vi "ArmPathPlanPreview.vi"(0 "RobotDimensions":T2, 2 "AvoidancePolygon":T6, 3 "Arm Pass Through Params":T1) -> (5 "Shoulder Path":T4[](array[typedef]) {"Time (ms)" items=["TrajectoryDuration_0ms"=0, "TrajectoryDuration_5ms"=5, "TrajectoryDuration_10ms"=10, "TrajectoryDuration_20ms"=20, "TrajectoryDuration_30ms"=30, "TrajectoryDuration_40ms"=40, "TrajectoryDuration_50ms"=50, "TrajectoryDuration_100ms"=100]}, 6 "Extension Path":T4[](array[typedef]) {"Time (ms)" items=["TrajectoryDuration_0ms"=0, "TrajectoryDuration_5ms"=5, "TrajectoryDuration_10ms"=10, "TrajectoryDuration_20ms"=20, "TrajectoryDuration_30ms"=30, "TrajectoryDuration_40ms"=40, "TrajectoryDuration_50ms"=50, "TrajectoryDuration_100ms"=100]}, 7 "Wrist Path":T4[](array[typedef]) {"Time (ms)" items=["TrajectoryDuration_0ms"=0, "TrajectoryDuration_5ms"=5, "TrajectoryDuration_10ms"=10, "TrajectoryDuration_20ms"=20, "TrajectoryDuration_30ms"=30, "TrajectoryDuration_40ms"=40, "TrajectoryDuration_50ms"=50, "TrajectoryDuration_100ms"=100]}, 8 "Go":bool)   [LabVIEW 2018]
uses:
  TypeDefs/ArmAbsolutePosition.ctl
  General/MotionProfiling/TypeDefs/MotionProfileGeneratorParams.ctl
  <vilib>/Rock Robotics/WPI/ThirdParty/Phoenix-LabVIEW/Motor Controller/Controls/CTRE_Phoenix_MotorControl_TrajectoryPointTimeDur.ctl
  General/MotionProfiling/TypeDefs/TrajectoryPoint.ctl
  ArgosLib/Path Planning/TypeDefs/Polygon2D.ctl
  ArgosLib/Path Planning/TypeDefs/Point2D.ctl
  TypeDefs/ConfigComponents/Config_Dimensions.ctl
  TypeDefs/ArmPassThroughParams.ctl
  ArgosLib/Signal Processing/TypeDefs/EdgeDetector_Type.ctl
  ArgosLib/ArgosLib.lvlib
panel:
  out "Wrist Path Graph":T3(graph)
  out "Shoulder Path Graph":T3(graph)
  in  "Preview?":bool
  in  "Send Path Plan":bool
  out "Extension Path Graph":T3(graph)
  in  "Reverse Direction":bool
  in  "MotionProfileGeneratorParameters":T8={"Trajectory Point Interval (ms)"=40, "Maximum Travel Speed (units/s)"=20.0, "Velocity Ramp Time (ms)"=400.0, "Acceleration Ramp Time (ms)"=200.0} {"Acceleration Ramp Time (ms)" min=1.0; "Velocity Ramp Time (ms)" min=1.0; "Maximum Travel Speed (units/s)" min=0.0; "Trajectory Point Interval (ms)" items=["TrajectoryDuration_0ms"=0, "TrajectoryDuration_5ms"=5, "TrajectoryDuration_10ms"=10, "TrajectoryDuration_20ms"=20, "TrajectoryDuration_30ms"=30, "TrajectoryDuration_40ms"=40, "TrajectoryDuration_50ms"=50, "TrajectoryDuration_100ms"=100]}
  in  "EndPoint":T9={"X (in)"=-21.5, "Y (in)"=0.0, "Wrist (rad)"=-1.57}
  in  "StartPoint":T9={"X (in)"=21.5, "Y (in)"=0.0, "Wrist (rad)"=1.57}
  in  "PathPointSpacing (in)":dbl=0.25
  in  "MaxArmLength":dbl=35.0
  in  "MinArmLength":dbl=17.0
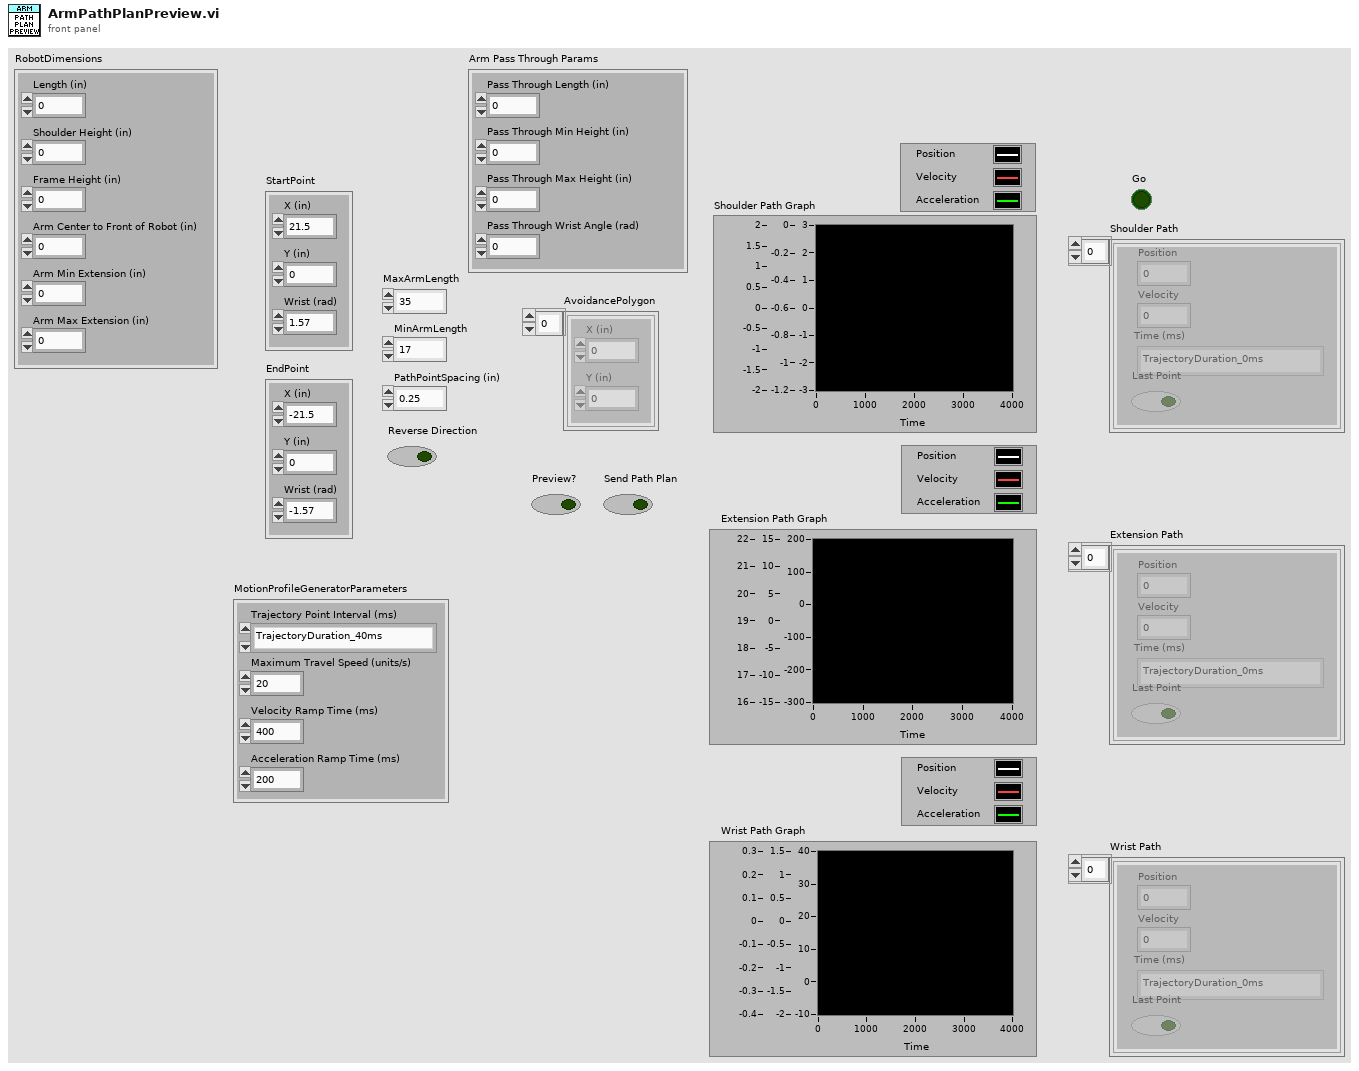
[diagram p1: front panel]
types:
  T1 = typedef "ArmPassThroughParams.ctl" = cluster{"Pass Through Length (in)":dbl, "Pass Through Min Height (in)":dbl, "Pass Through Max Height (in)":dbl, "Pass Through Wrist Angle (rad)":dbl}
  T2 = typedef "Config_Dimensions.ctl" = cluster{"Length (in)":dbl, "Shoulder Height (in)":dbl, "Frame Height (in)":dbl, "Arm Center to Front of Robot (in)":dbl, "Arm Min Extension (in)":dbl, "Arm Max Extension (in)":dbl}
  T3 = cluster{dbl, "Trajectory Point Interval (ms)":i32, dbl[][]}
  T4 = typedef "TrajectoryPoint.ctl" = cluster{"Position ":dbl, "Velocity ":dbl, "Time (ms)":T5, "Last Point":bool}
  T5 = typedef "CTRE_Phoenix_MotorControl_TrajectoryPointTimeDur.ctl" = i32
  T6 = typedef "ArgosLib.lvlib/Polygon2D.ctl" = T7[]
  T7 = typedef "ArgosLib.lvlib/Point2D.ctl" = cluster{"X (in)":dbl, "Y (in)":dbl}
  T8 = typedef "MotionProfileGeneratorParams.ctl" = cluster{"Trajectory Point Interval (ms)":T5, "Maximum Travel Speed (units/s)":dbl, "Velocity Ramp Time (ms)":dbl, "Acceleration Ramp Time (ms)":dbl}
  T9 = typedef "ArmAbsolutePosition.ctl" = cluster{"X (in)":dbl, "Y (in)":dbl, "Wrist (rad)":dbl}
  T10 = typedef "ArgosLib.lvlib/EdgeDetector_Type.ctl" = enum16{"RisingEdge", "FallingEdge", "Both"}
  T11 = cluster{dbl, "Trajectory Point Interval (ms)":T5, dbl[][]}
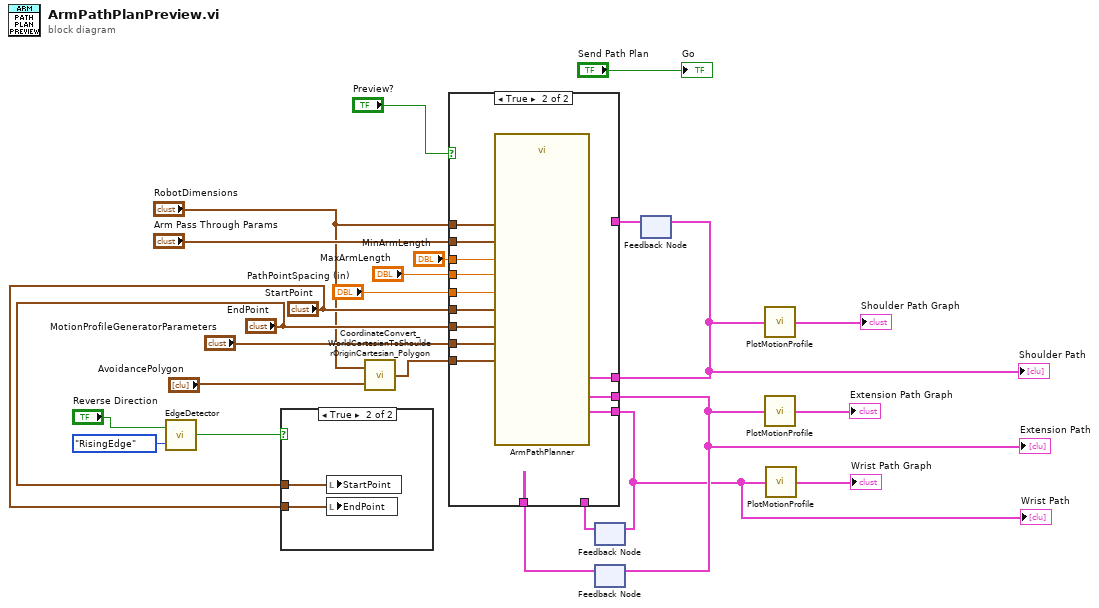
[diagram p0: block diagram]
diagram:
  n1 = call "EdgeDetector.vi"("DetectorType"=EdgeDetector_Type."RisingEdge", "Input"="Reverse Direction") -> ("Edge"=w20:bool)
  n2 = case shown="True" w20 {
    tunnel: "StartPoint" -> [_ w26]
    tunnel: "EndPoint" -> [_ w25]
    frame False {
    }
    frame True {
      n3 = local write "StartPoint"(w25) -> ()
      n4 = local write "EndPoint"(w26) -> ()
    }
  }
  n5 = call "CoordinateConvert_WorldCartesianToShoulderOriginCartesian_Polygon.vi"("ArmPositionIn"="AvoidancePolygon", "RobotDimensions"="RobotDimensions") -> ("ArmPositionRelativeToShoulder"=w2:T6)
  n6 = feedback #1() -> (w4:T4[])  [unwired: 1 in]
  n7 = feedback #2() -> (w11:T4[])  [unwired: 1 in]
  n8 = feedback #3() -> (w9:T4[])  [unwired: 1 in]
  n9 = case shown="True" "Preview?" {
    tunnel: "MinArmLength" -> [_ w41]
    tunnel: "MaxArmLength" -> [_ w40]
    tunnel: "PathPointSpacing (in)" -> [_ w39]
    tunnel: "MotionProfileGeneratorParameters" -> [_ w38]
    tunnel: "StartPoint" -> [_ w37]
    tunnel: "EndPoint" -> [_ w36]
    tunnel: [w28 w34] -> w10
    tunnel: [w29 w35] -> w12
    tunnel: w11 -> [w29 _]
    tunnel: w9 -> [w28 _]
    tunnel: w2 -> [_ w33]
    tunnel: [w27 w32] -> w5
    tunnel: w4 -> [w27 _]
    tunnel: "RobotDimensions" -> [_ w31]
    tunnel: "Arm Pass Through Params" -> [_ w30]
    frame False {
    }
    frame True {
      n10 = call "ArmPathPlanner.vi"("StartPoint"=w37, "EndPoint"=w36, "PathPointSpacing (in)"=w39, "MinArmLength"=w41, "MaxArmLength"=w40, "AvoidancePolygon"=w33, "RobotDimensions"=w31, "MotionProfileGeneratorParameters"=w38, "Arm Pass Through Params"=w30) -> ("ShoulderPath"=w34:T4[], "ExtendPath"=w35:T4[], "WristPath"=w32:T4[])  [unwired: 6 in, 2 out]
    }
  }
  "Shoulder Path" <- w10
  "Extension Path" <- w12
  "Wrist Path" <- w5
  n11 = feedback-in #1(w5) -> ()
  n12 = feedback-in #2(w12) -> ()
  n13 = feedback-in #3(w10) -> ()
  n14 = call "PlotMotionProfile.vi"("Trajectory Points"=w10) -> ("MotionProfileGraph"=→"Shoulder Path Graph":T11)
  n15 = call "PlotMotionProfile.vi"("Trajectory Points"=w12) -> ("MotionProfileGraph"=→"Extension Path Graph":T11)
  n16 = call "PlotMotionProfile.vi"("Trajectory Points"=w5) -> ("MotionProfileGraph"=→"Wrist Path Graph":T11)
  "Go" <- "Send Path Plan"
